vi "VISA_Keithley2230G_ConfigureInstrument_V1.vi"(0 "VISA resource name":refnum<visa-resource-name>, 1 "VISAPowerInfoInputArray":T2(array[cluster]), 2 "Input Array (Voltage,Current_Limit)":dbl[][](array[numeric]), 3 "Combination Scheme":u16(ring) items=["OFF", "SERIES", "PARALLEL"], 4 "Which Channels to Parallelize":u16(ring) items=["I1+I2", "ALL", "I2+I3"], 5 "error in":errorcluster, 6 "POWER STATUS IN":bool) -> (12 "POWER STATUS OUT":bool, 15 "VISAPowerInfoOutputArray":T2(array[cluster]), 17 "Configuration Echo":string, 18 "Parameter Configuration Echo":string[][](array[string]), 19 "error out":errorcluster)   [LabVIEW 2019]
panel:
  out "Cluster 2":T1
  in  "Cluster":T1
  out "VISAPowerInformationClusterOutput":T3(array[cluster])
  in  "VISAPowerInformationClusterInput":T3(array[cluster])
  in  "Channel Names":string[](array[string])
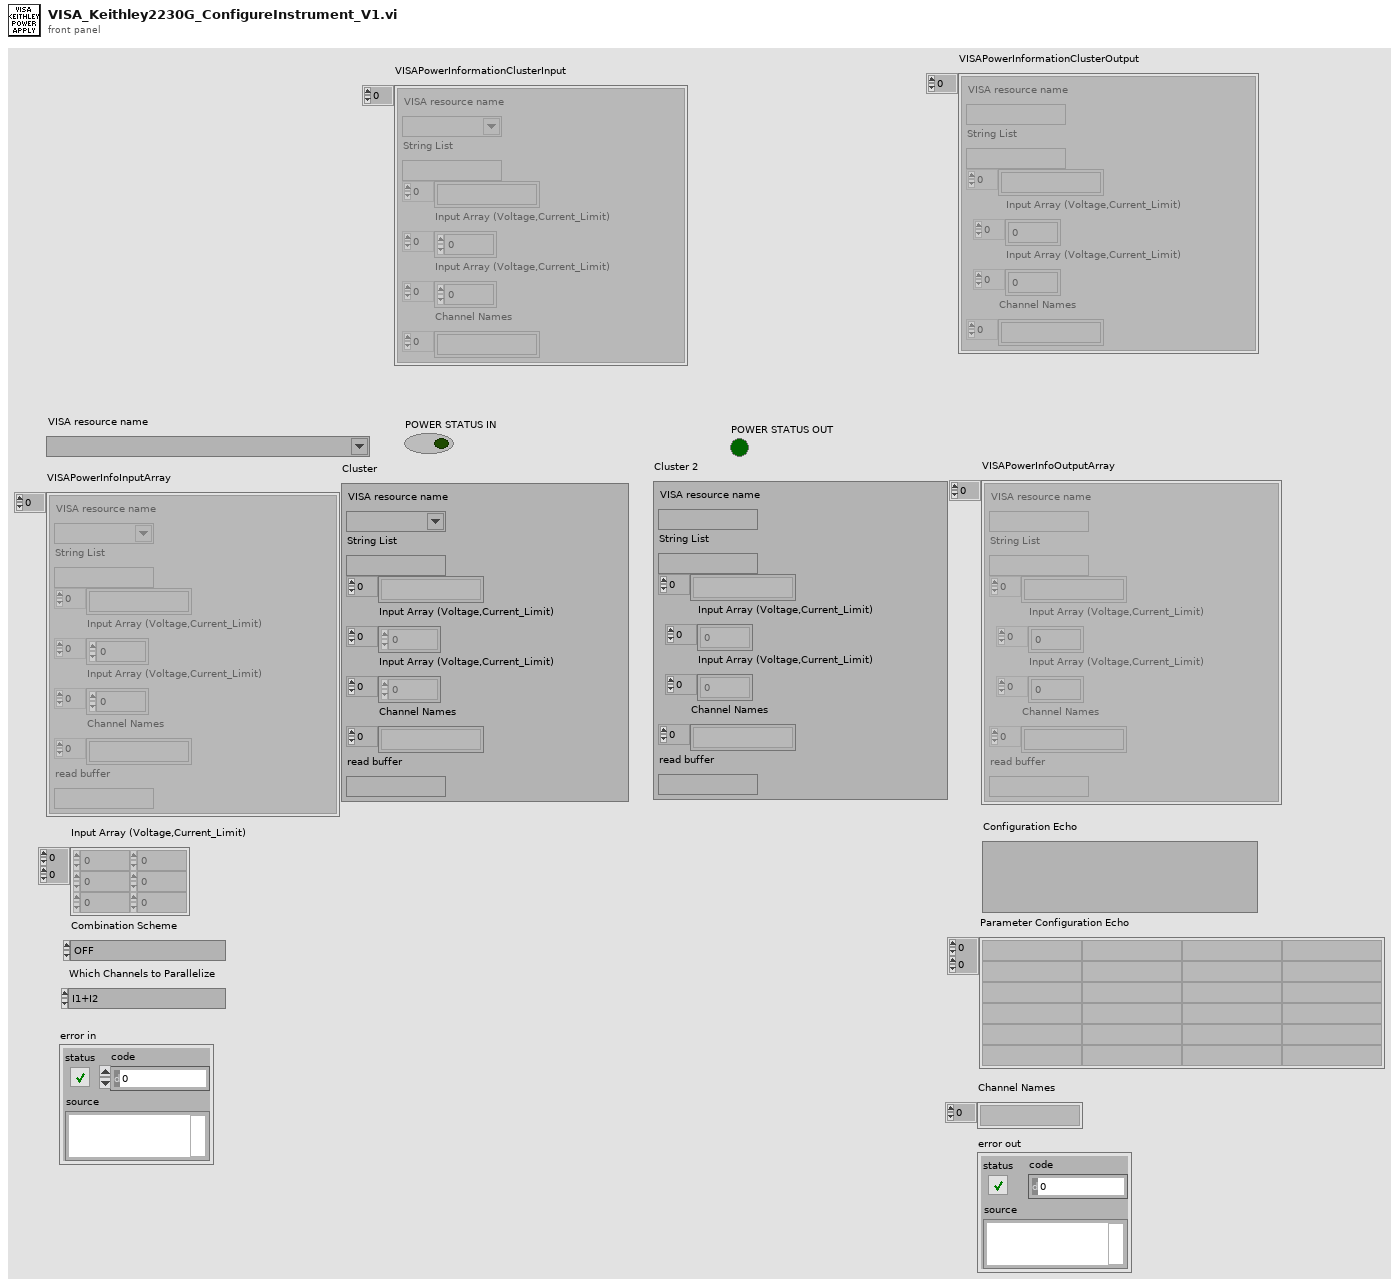
[diagram p1: front panel]
types:
  T1 = cluster{"VISA resource name":refnum<visa-resource-name>, "String List":string, string[], "Input Array (Voltage,Current_Limit)":dbl[], "Input Array (Voltage,Current_Limit)":dbl[], "Channel Names":string[], "read buffer":string}
  T2 = cluster{"VISA resource name":refnum<visa-resource-name>, "String List":string, string[], "Input Array (Voltage,Current_Limit)":dbl[], "Input Array (Voltage,Current_Limit)":dbl[], "Channel Names":string[], "read buffer":string}[]
  T3 = cluster{"VISA resource name":refnum<visa-resource-name>, "String List":string, string[], "Input Array (Voltage,Current_Limit)":dbl[], "Input Array (Voltage,Current_Limit)":dbl[], "Channel Names":string[]}[]
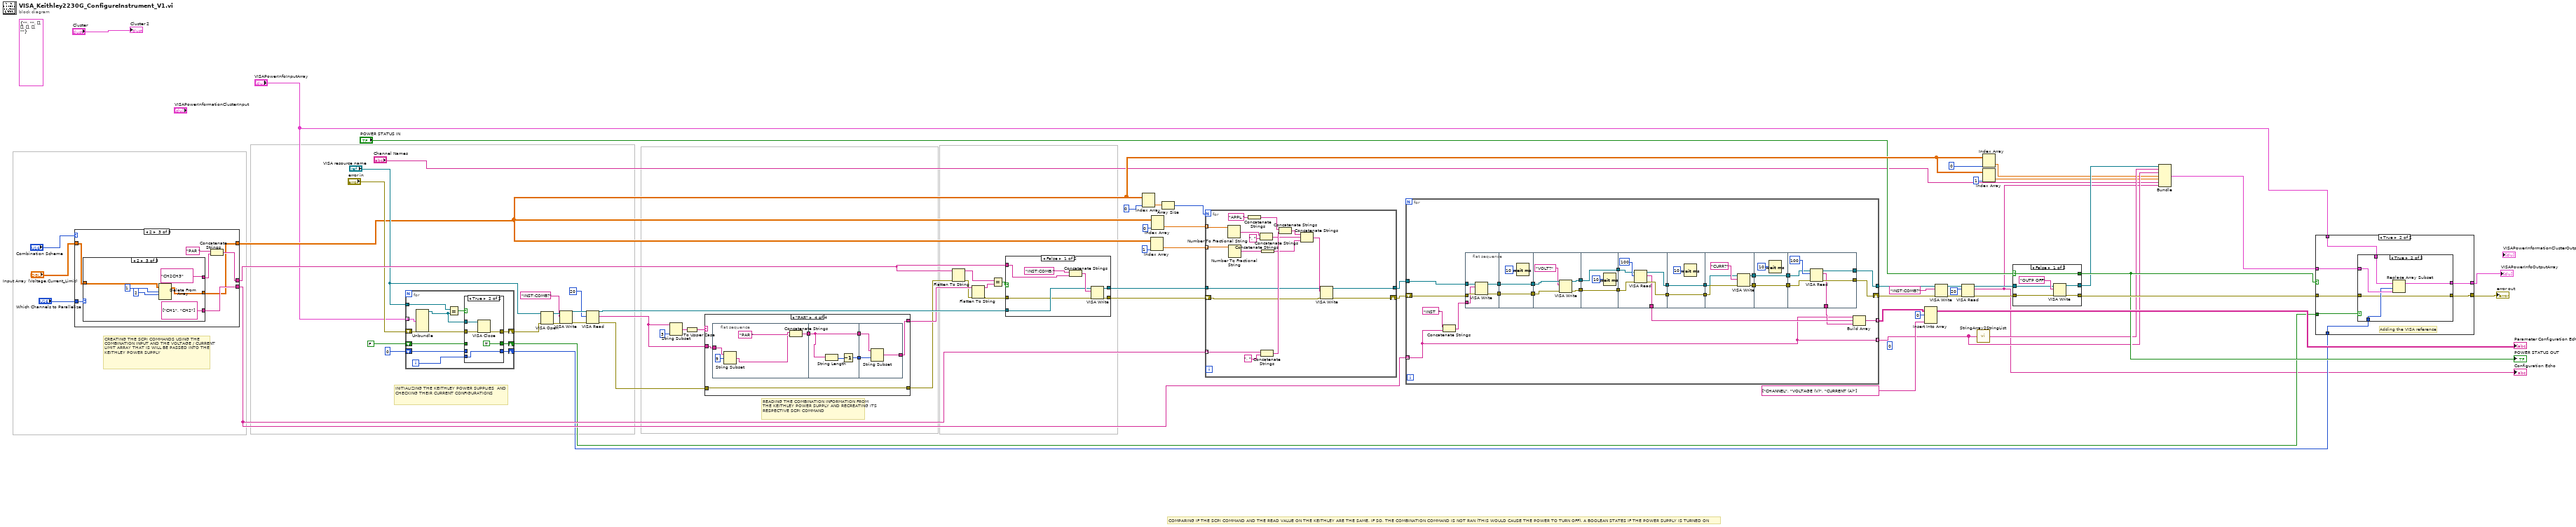
[diagram p0: block diagram]
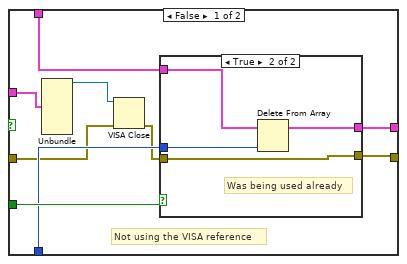
[diagram p2: hidden frame]
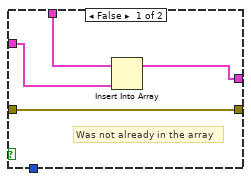
[diagram p4: hidden frame]
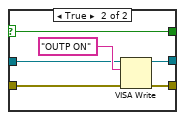
[diagram p5: hidden frame]
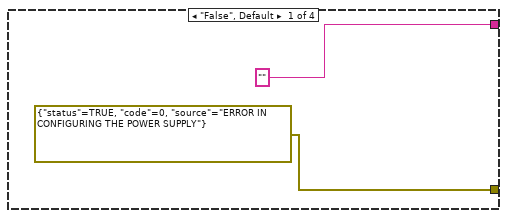
[diagram p8: hidden frame]
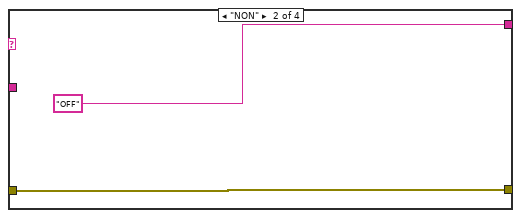
[diagram p9: hidden frame]
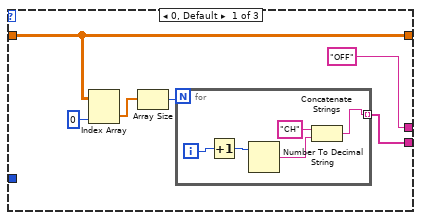
[diagram p11: hidden frame]
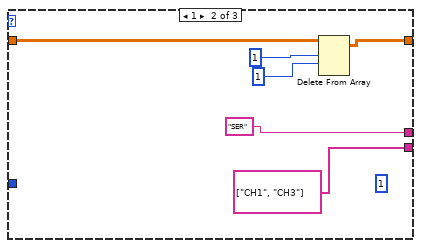
[diagram p12: hidden frame]
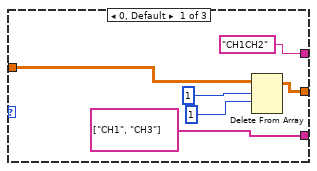
[diagram p13: hidden frame]
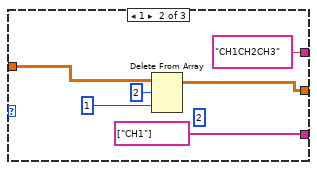
[diagram p14: hidden frame]
diagram:
  (unwired) T1 {"VISA resource name"="", "String List"="", [], "Input Array (Voltage,Current_Limit)"=[], "Input Array (Voltage,Current_Limit)"=[], "Channel Names"=[], "read buffer"=""}
  (unwired) 0
  # "COMPARING IF THE SCPI COMMAND AND THE READ VALUE ON THE KEITHLEY ARE THE SAME. IF SO, THE COMBINATION COMMAND IS NOT RAN (THIS WOULD CAUSE THE POWER TO TURN OFF). A BOOLEAN STATES IF THE POWER SUPPLY IS TURNED ON"
  # "READING THE COMBINATION INFORMATION FROM THE KEITHLEY POWER SUPPLY AND RECREATING ITS RESPECTIVE SCPI COMMAND"
  # "CREATING THE SCPI COMMANDS USING THE COMBINATION INPUT AND THE VOLTAGE / CURRENT LIMIT ARRAY THAT IS WILL BE PASSED INTO THE KEITHLEY POWER SUPPLY"
  # "INITIALIZING THE KEITHLEY POWER SUPPLIES  AND CHECKING THEIR CURRENT CONFIGURATIONS"
  n1 = case shown="2" "Combination Scheme" {
    tunnel: ["OFF" "SER" w93] -> w45
    tunnel: "Which Channels to Parallelize" -> [_ _ w96]
    tunnel: "Input Array (Voltage,Current_Limit)" -> [w77 w87 w91]
    tunnel: [w77 w84 w90] -> w21
    tunnel: [w73 string[] ["CH1", "CH3"] w92] -> w30
    frame 0, Default {
      n2 = Index Array(array=w77, index (col)=0 ("disabled index (col)")) -> (element=w76:dbl[])  [unwired: 1 in]
      n3 = Array Size(array=w76) -> (size(s)=w74:i32)
      n4 = for {
        N: w74 -> [_]
        tunnel: [w79] -> w73 mode=indexing
        i -> [w82]
        n5 = Increment(x=w82) -> (x+1=w83:i32)
        n6 = Number To Decimal String(number=w83) -> (decimal integer string=w81:string)  [unwired: 1 in]
        n7 = Concatenate Strings("CH" ("string"), w81) -> (w79:string)
      }
    }
    frame 1 {
      (unwired) 1
      n8 = Delete From Array(array=w87, length=1, index (row)=1) -> (array with subset deleted=w84:dbl[][])  [unwired: 1 in, 1 out]
    }
    frame 2 {
      n9 = case shown="2" w96 {
        tunnel: ["CH1CH2" "CH1CH2CH3" "CH2CH3"] -> w94
        tunnel: [string[] ["CH1", "CH3"] string[] ["CH1"] string[] ["CH1", "CH2"]] -> w92
        tunnel: w91 -> [w98 w106 w110]
        tunnel: [w97 w103 w111] -> w90
        frame 0, Default {
          n10 = Delete From Array(array=w98, length=1, index (row)=1) -> (array with subset deleted=w97:dbl[][])  [unwired: 1 in, 1 out]
        }
        frame 1 {
          (unwired) 2 ("index (row)")
          n11 = Delete From Array(array=w106, length=2, index (row)=1) -> (array with subset deleted=w103:dbl[][])  [unwired: 1 in, 1 out]
        }
        frame 2 {
          n12 = Delete From Array(array=w110, length=1, index (row)=2) -> (array with subset deleted=w111:dbl[][])  [unwired: 1 in, 1 out]
        }
      }
      n13 = Concatenate Strings("PAR ", w94) -> (w93:string)
    }
  }
  n14 = for {
    tunnel: "VISA resource name" -> [w119]
    shift-right: [w123] -> w12
    shift-left: FALSE -> [w124]
    shift-right: [w120] -> w11
    shift-left: 0 -> [w121]
    shift-right: [w118] -> w24
    shift-left: "error in" -> [w117]
    tunnel: "VISAPowerInfoInputArray" -> [w116] mode=indexing
    i -> [w122]
    n15 = Unbundle(w116) -> ("VISA resource name"=w115:refnum<visa-resource-name>)  [unwired: 6 out]
    n16 = Equal?(x=w119, y=w115) -> (x = y?=w125:bool)
    n17 = case shown="True" w125 {
      tunnel: w124 -> [w128 _]
      tunnel: [w128 TRUE] -> w123
      tunnel: w122 -> [_ w132]
      tunnel: w121 -> [w127 _]
      tunnel: [w127 w132] -> w120
      tunnel: [w126 w131] -> w118
      tunnel: w117 -> [w126 w130]
      tunnel: w115 -> [_ w129]
      frame False {
      }
      frame True {
        n18 = VISA Close(VISA resource name=w129, error in (no error)=w130) -> (error out=w131:errorcluster)
      }
    }
  }
  n19 = VISA Open(error in (no error)=w24, VISA resource name="VISA resource name") -> (VISA resource name=w60:refnum<visa-resource-name>, error out=w59:errorcluster)  [unwired: 3 in]
  n20 = VISA Write(VISA resource name=w60, write buffer="INST:COMB?", error in (no error)=w59) -> (VISA resource name out=w58:refnum<visa-resource-name>, error out=w57:errorcluster)  [unwired: 1 out]
  n21 = VISA Read(VISA resource name=w58, byte count=u32 20, error in (no error)=w57) -> (VISA resource name out=w54:refnum<visa-resource-name>, read buffer=w43:string, error out=w42:errorcluster)  [unwired: 1 out]
  n22 = String Subset(string=w43, length (rest)=3 ("length (rest)")) -> (substring=w51:string)  [unwired: 1 in]
  n23 = To Upper Case(1:w51) -> (0:w52:string)
  n24 = case shown="\"PAR\"" w52 {
    selector: w52 -> [_ _ w138 _]
    tunnel: ["" "OFF" w138 w140] -> w50
    tunnel: w43 -> [_ _ _ w145]
    tunnel: w42 -> [_ w136 w139 w144]
    tunnel: [errorcluster {"status"=TRUE, "code"=0, "source"="ERROR IN CONFIGURING THE POWER SUPPLY"} ("error out") w136 w139 w144] -> w41
    frame "False", Default {
    }
    frame "NON" {
    }
    frame "SER" {
    }
    frame "PAR" {
      n25 = flat-sequence {
        tunnel: w145 -> [w149]
        tunnel: [w146] -> w143
        tunnel: w143 -> [w152]
        tunnel: [w152] -> w142
        tunnel: [w151] -> w141
        tunnel: w142 -> [w155]
        tunnel: w141 -> [w156]
        tunnel: [w154] -> w140
        frame #0 {
          n26 = String Subset(string=w149, offset (0)=9) -> (substring=w147:string)  [unwired: 1 in]
          n27 = Concatenate Strings("PAR ", w147) -> (w146:string)
        }
        frame #1 {
          n28 = String Length(string=w152) -> (length=w153:i32)
          n29 = Decrement(x=w153) -> (x-1=w151:i32)
        }
        frame #2 {
          n30 = String Subset(string=w155, length (rest)=w156) -> (substring=w154:string)  [unwired: 1 in]
        }
      }
    }
  }
  n31 = Flatten To String(anything=w45, error in (no error)=w41) -> (data string=w48:string, error out=w47:errorcluster)  [unwired: 2 in, 1 out]
  n32 = Flatten To String(anything=w50, error in (no error)=w47) -> (data string=w49:string, error out=w46:errorcluster)  [unwired: 2 in, 1 out]
  n33 = Equal?(x=w48, y=w49) -> (x = y?=w44:bool)
  n34 = case shown="False" w44 {
    tunnel: [w161 w165] -> w63
    tunnel: [w160 w164] -> w62
    tunnel: w54 -> [w159 w165]
    tunnel: w46 -> [w158 w164]
    tunnel: w45 -> [w157 _]
    frame False {
      n35 = Concatenate Strings("INST:COMB:" ("string"), w157) -> (w163:string)
      n36 = VISA Write(VISA resource name=w159, write buffer=w163, error in (no error)=w158) -> (VISA resource name out=w161:refnum<visa-resource-name>, error out=w160:errorcluster)  [unwired: 1 out]
    }
    frame True {
    }
  }
  n37 = Index Array(array=w21, index (col)=0 ("disabled index (col)")) -> (element=w71:dbl[])  [unwired: 1 in]
  n38 = Index Array(array=w21, index (col)=1 ("disabled index (col)")) -> (element=w66:dbl[])  [unwired: 1 in]
  n39 = Index Array(array=w21, index (col)=0 ("disabled index (col)")) -> (element=w67:dbl[])  [unwired: 1 in]
  n40 = Array Size(array=w71) -> (size(s)=w70:i32)
  n41 = for {
    N: w70 -> [_]
    tunnel: w63 -> [w168]
    tunnel: w67 -> [w178] mode=indexing
    tunnel: w66 -> [w177] mode=indexing
    tunnel: [w183] -> w36
    shift-right: [w182] -> w35
    shift-left: w62 -> [w167]
    tunnel: w30 -> [w166] mode=indexing
    n42 = Number To Fractional String(number=w178) -> (F-format string=w176:string)  [unwired: 3 in]
    n43 = Number To Fractional String(number=w177) -> (F-format string=w174:string)  [unwired: 3 in]
    n44 = Concatenate Strings("APPL " ("string")) -> (w179:string)
    n45 = Concatenate Strings(w176, ", " ("string")) -> (w172:string)
    n46 = Concatenate Strings(w166, ", " ("string")) -> (w180:string)
    n47 = Concatenate Strings(w174) -> (w171:string)
    n48 = Concatenate Strings(w179, w180) -> (w173:string)
    n49 = Concatenate Strings(w173, w172, w171) -> (w170:string)
    n50 = VISA Write(VISA resource name=w168, write buffer=w170, error in (no error)=w167) -> (VISA resource name out=w183:refnum<visa-resource-name>, error out=w182:errorcluster)  [unwired: 1 out]
  }
  n51 = for {
    tunnel: w36 -> [w209]
    tunnel: [w201] -> w33
    shift-right: [w203] -> w34
    shift-left: w35 -> [w208]
    tunnel: [w205] -> w29 mode=indexing
    tunnel: w30 -> [w184] mode=indexing
    tunnel: [w184] -> w8 mode=indexing
    n52 = Concatenate Strings("INST  " ("string"), w184) -> (w206:string)
    n53 = flat-sequence {
      tunnel: w209 -> [w214]
      tunnel: w208 -> [w213]
      tunnel: w206 -> [w212]
      tunnel: [w211] -> w188
      tunnel: [w210] -> w186
      tunnel: w188 -> [w217]
      tunnel: [w217] -> w187
      tunnel: w186 -> [w216]
      tunnel: [w216] -> w185
      tunnel: w187 -> [w221]
      tunnel: w185 -> [w222]
      tunnel: [w220] -> w200
      tunnel: [w219] -> w198
      tunnel: w200 -> [w225]
      tunnel: [w225] -> w199
      tunnel: w198 -> [w224]
      tunnel: [w224] -> w197
      tunnel: w199 -> [w231]
      tunnel: w197 -> [w229]
      tunnel: [w227] -> w204
      tunnel: [w228] -> w196
      tunnel: [w226] -> w194
      tunnel: w196 -> [w234]
      tunnel: [w234] -> w195
      tunnel: w194 -> [w233]
      tunnel: [w233] -> w193
      tunnel: w195 -> [w239]
      tunnel: w193 -> [w237]
      tunnel: [w236] -> w192
      tunnel: [w235] -> w190
      tunnel: w192 -> [w240]
      tunnel: [w240] -> w191
      tunnel: w190 -> [w242]
      tunnel: [w242] -> w189
      tunnel: w191 -> [w248]
      tunnel: w189 -> [w246]
      tunnel: [w245] -> w203
      tunnel: [w244] -> w202
      tunnel: [w243] -> w201
      frame #0 {
        n54 = VISA Write(VISA resource name=w214, write buffer=w212, error in (no error)=w213) -> (VISA resource name out=w211:refnum<visa-resource-name>, error out=w210:errorcluster)  [unwired: 1 out]
      }
      frame #1 {
        n55 = Wait (ms)(milliseconds to wait=u32 10) -> ()  [unwired: 1 out]
      }
      frame #2 {
        n56 = VISA Write(VISA resource name=w221, write buffer="VOLT?", error in (no error)=w222) -> (VISA resource name out=w219:refnum<visa-resource-name>, error out=w220:errorcluster)  [unwired: 1 out]
      }
      frame #3 {
        n57 = Wait (ms)(milliseconds to wait=u32 10) -> ()  [unwired: 1 out]
      }
      frame #4 {
        n58 = VISA Read(VISA resource name=w229, byte count=u32 100, error in (no error)=w231) -> (VISA resource name out=w226:refnum<visa-resource-name>, read buffer=w227:string, error out=w228:errorcluster)  [unwired: 1 out]
      }
      frame #5 {
        n59 = Wait (ms)(milliseconds to wait=u32 10) -> ()  [unwired: 1 out]
      }
      frame #6 {
        n60 = VISA Write(VISA resource name=w237, write buffer="CURR?", error in (no error)=w239) -> (VISA resource name out=w235:refnum<visa-resource-name>, error out=w236:errorcluster)  [unwired: 1 out]
      }
      frame #7 {
        n61 = Wait (ms)(milliseconds to wait=u32 10) -> ()  [unwired: 1 out]
      }
      frame #8 {
        n62 = VISA Read(VISA resource name=w246, byte count=u32 100, error in (no error)=w248) -> (VISA resource name out=w243:refnum<visa-resource-name>, read buffer=w244:string, error out=w245:errorcluster)  [unwired: 1 out]
      }
    }
    n63 = Build Array(w184, w204, w202) -> (w205:string[])
  }
  n64 = Insert Into Array(array=w29, index (row)=0, new element=string[] ["CHANNEL", "VOLTAGE (V)", "CURRENT (A)"] ("new element/subarray")) -> (→"Parameter Configuration Echo":string[][])  [unwired: 1 in]
  n65 = VISA Write(VISA resource name=w33, write buffer="INST:COMB?", error in (no error)=w34) -> (VISA resource name out=w40:refnum<visa-resource-name>, error out=w39:errorcluster)  [unwired: 1 out]
  n66 = VISA Read(VISA resource name=w40, byte count=u32 20, error in (no error)=w39) -> (VISA resource name out=w19:refnum<visa-resource-name>, read buffer=w3:string, error out=w18:errorcluster)  [unwired: 1 out]
  "Configuration Echo" <- w3
  n67 = call "StringArray2StringList.vi"("String Array"=w8) -> ("String List"=w9:string)
  n68 = Index Array(array=w21, index (col)=0 ("disabled index (col)")) -> (element=w7:dbl[])  [unwired: 1 in]
  n69 = Index Array(array=w21, index (col)=1 ("disabled index (col)")) -> (element=w6:dbl[])  [unwired: 1 in]
  n70 = case shown="False" "POWER STATUS IN" {
    selector: "POWER STATUS IN" -> [w249 w255]
    tunnel: w19 -> [w252 w259]
    tunnel: w18 -> [w253 w258]
    tunnel: [w251 w257] -> w15
    tunnel: [w250 w256] -> w10
    tunnel: [w249 w255] -> w14
    frame False {
      n71 = VISA Write(VISA resource name=w252, write buffer="OUTP OFF", error in (no error)=w253) -> (VISA resource name out=w250:refnum<visa-resource-name>, error out=w251:errorcluster)  [unwired: 1 out]
    }
    frame True {
      n72 = VISA Write(VISA resource name=w259, write buffer="OUTP ON", error in (no error)=w258) -> (VISA resource name out=w256:refnum<visa-resource-name>, error out=w257:errorcluster)  [unwired: 1 out]
    }
  }
  "POWER STATUS OUT" <- w14
  n73 = Bundle("VISA resource name"=w10, "String List"=w9, w8, "Input Array (Voltage,Current_Limit)"=w7, "Input Array (Voltage,Current_Limit)"=w6, "Channel Names"="Channel Names", "read buffer"=w3) -> (w13:T1)  [unwired: 1 in]
  n74 = case shown="True" w14 {
    tunnel: [w265 w278] -> w16
    tunnel: w15 -> [w263 w277]
    tunnel: w13 -> [w264 w282]
    tunnel: w12 -> [w269 w281]
    tunnel: w11 -> [w267 w280]
    tunnel: "VISAPowerInfoInputArray" -> [w268 w279]
    tunnel: [w266 w276] -> w2
    frame False {
      # "Not using the VISA reference"
      n75 = Unbundle(w264) -> ("VISA resource name"=w261:refnum<visa-resource-name>)  [unwired: 6 out]
      n76 = VISA Close(VISA resource name=w261, error in (no error)=w263) -> (error out=w262:errorcluster)
      n77 = case shown="True" w269 {
        tunnel: w268 -> [w271 w275]
        tunnel: w267 -> [_ w274]
        tunnel: [w271 w273] -> w266
        tunnel: [w270 w272] -> w265
        tunnel: w262 -> [w270 w272]
        frame False {
          # "Not being used"
        }
        frame True {
          # "Was being used already"
          n78 = Delete From Array(array=w275, index=w274) -> (array with subset deleted=w273:T2)  [unwired: 1 in, 1 out]
        }
      }
    }
    frame True {
      # "Adding the VISA reference"
      n79 = case shown="True" w281 {
        tunnel: w282 -> [w285 w291]
        tunnel: w280 -> [_ w289]
        tunnel: w279 -> [w286 w290]
        tunnel: [w284 w288] -> w278
        tunnel: w277 -> [w284 w288]
        tunnel: [w283 w287] -> w276
        frame False {
          # "Was not already in the array"
          n80 = Insert Into Array(array=w286, new element=w285) -> (w283:T2)  [unwired: 1 in]
        }
        frame True {
          n81 = Replace Array Subset(array=w290, new element=w291, index=w289) -> (w287:T2)
        }
      }
    }
  }
  "error out" <- w16
  "VISAPowerInfoOutputArray" <- w2
  "Cluster 2" <- "Cluster"
